vi "FileLoad.vi"(7 "측정거리":dbl, 8 "노이즈 수량":u16=280, 9 "거리 해상도":sgl, 10 "스톡스 데이터 경로 문자열":string, 11 "안티스톡스 데이터 경로 문자열":string) -> (0 "스톡스 인덱스":i32, 1 "안티스톡스 인덱스":i32, 2 "스톡스 배열":dbl[](array[numeric]) caption="스톡스 데이터 배열", 3 "안티스톡스 배열":dbl[](array[numeric]) caption="안티스톡스 데이터 배열", 4 "거리축 배열":dbl[](array[numeric]), 5 "데이터 총량":u32, 6 "대기중":bool)   [LabVIEW 2020]
uses:
  <vilib>/Utility/error.llb/DialogType.ctl
panel:
  out "안티스톡스 OffSet":bool
  out "스톡스 OffSet":bool
  out "안티스톡스 OffSet 평균":dbl
  out "스톡스 OffSet 평균":dbl
  out "OffSet 평균":bool
  out "안티스톡스 읽기 완료":bool caption="읽기완료"
  out "안티스톡스 데이터 경로":path
  out "스톡스 읽기 완료":bool caption="읽기완료"
  out "스톡스 데이터 경로":path
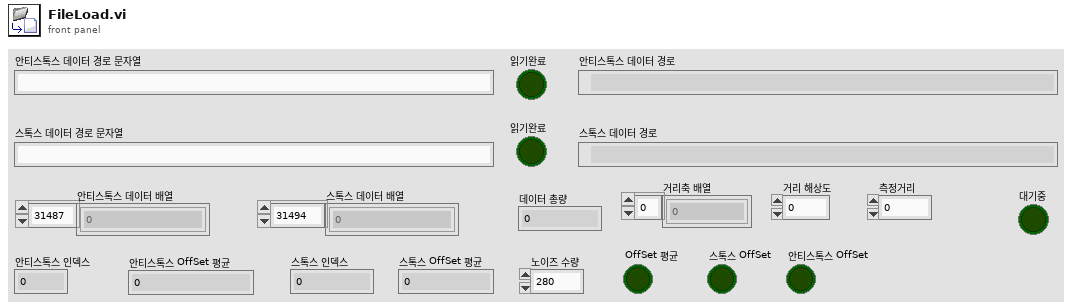
[diagram p1: front panel]
types:
  T1 = typedef "DialogType.ctl" = u16
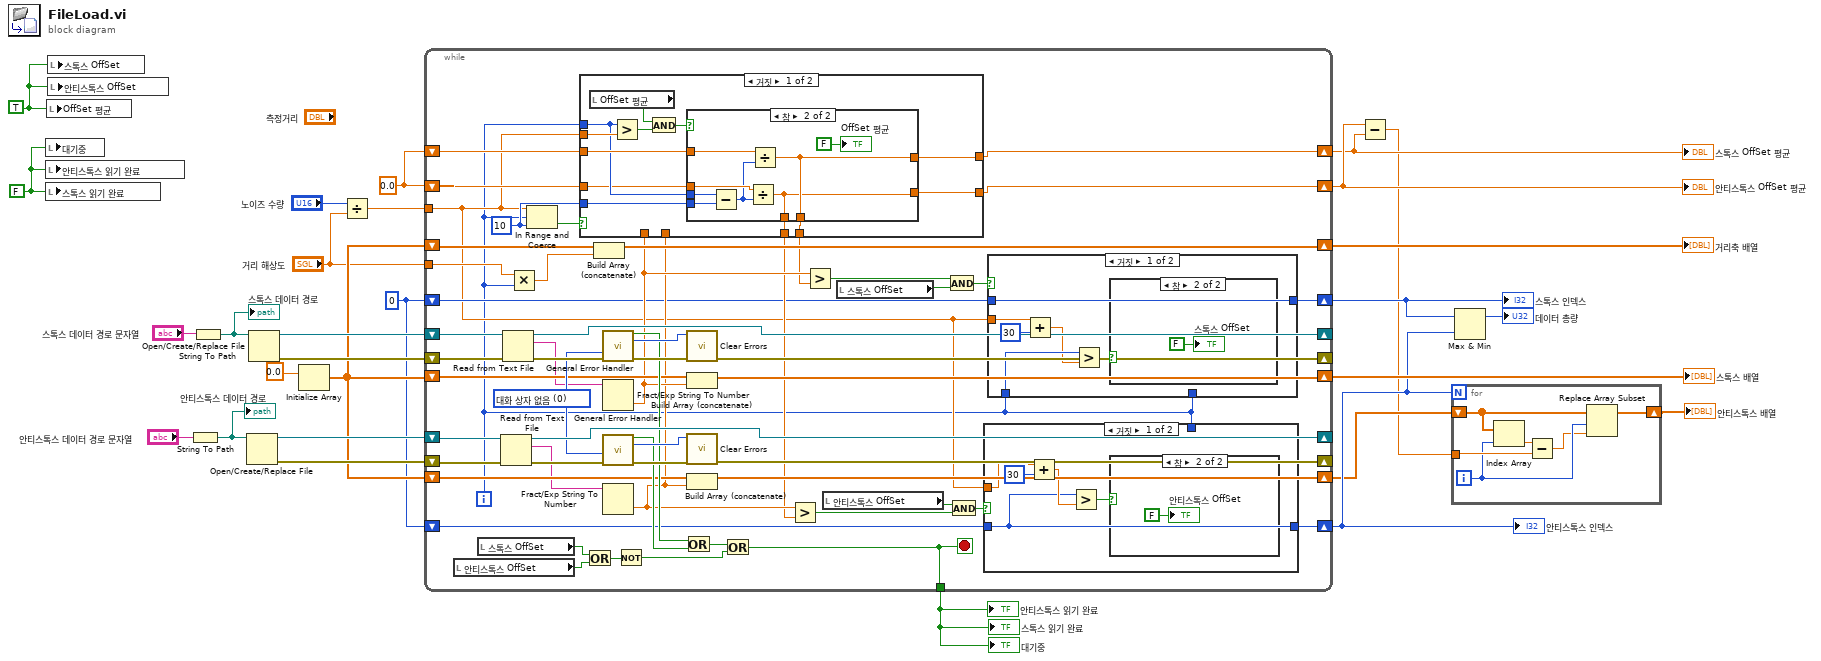
[diagram p0: block diagram]
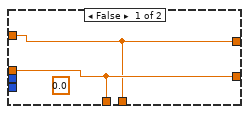
[diagram p6: hidden frame]
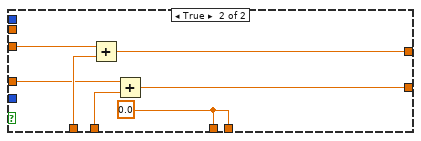
[diagram p7: hidden frame]
diagram:
  w13 = 0
  w12 = TRUE
  w14 = 0.0
  w15 = FALSE
  n1 = local write "대기중"(w15) -> ()
  n2 = local write "안티스톡스 읽기 완료"(w15) -> ()
  n3 = local write "스톡스 읽기 완료"(w15) -> ()
  n4 = local write "OffSet 평균"(w12) -> ()
  n5 = local write "스톡스 OffSet"(w12) -> ()
  n6 = local write "안티스톡스 OffSet"(w12) -> ()
  n7 = String To Path(string="안티스톡스 데이터 경로 문자열") -> (path=w23:path)
  "안티스톡스 데이터 경로" <- w23
  n8 = String To Path(string="스톡스 데이터 경로 문자열") -> (path=w24:path)
  "스톡스 데이터 경로" <- w24
  n9 = Open/Create/Replace File(file path (use dialog)=w23) -> (refnum out=w26:refnum<file>, error out=w25:errorcluster)  [unwired: 5 in, 1 out]
  n10 = Open/Create/Replace File(file path (use dialog)=w24) -> (refnum out=w28:refnum<file>, error out=w27:errorcluster)  [unwired: 5 in, 1 out]
  n11 = Initialize Array(0.0) -> (w17:dbl[])  [unwired: 1 in]
  n12 = Divide(x="노이즈 수량", y="거리 해상도") -> (x/y=w1:sgl)
  n13 = while {
    shift-right: [w78] -> _
    shift-left: w28 -> [w83]
    shift-right: [w79] -> _
    shift-left: w27 -> [w82]
    shift-right: [w70] -> _
    shift-left: w26 -> [w75]
    shift-right: [w71] -> _
    shift-left: w25 -> [w74]
    tunnel: [w30] -> w20
    shift-right: [w63] -> w18
    shift-left: w17 -> [w66]
    shift-right: [w64] -> w6
    shift-left: w17 -> [w65]
    tunnel: "거리 해상도" -> [w60]
    shift-right: [w58] -> w16
    shift-left: w17 -> [w59]
    tunnel: w1 -> [w37]
    shift-right: [w51] -> w9
    shift-left: w14 -> [w53]
    shift-right: [w54] -> w8
    shift-left: w14 -> [w56]
    shift-right: [w47] -> w11
    shift-left: w13 -> [w46]
    shift-right: [w44] -> w7
    shift-left: w13 -> [w45]
    i -> [w36]
    stop <- w30 stop-if-true
    w50 = 10 ("하위 리미트")
    w69 = T1 0 items=["대화 상자 없음", "확인 메시지", "메시지 지속 또는 정지", "확인 메시지 + 경고", "지속/정지 + 경고"] ("type of dialog (OK msg:1)")
    n14 = local read "안티스톡스 OffSet"() -> (w34:bool)
    n15 = local read "스톡스 OffSet"() -> (w35:bool)
    n16 = Read from Text File(file (use dialog)=w75, error in=w74) -> (refnum out=w70:refnum<file>, text=w61:string, error out=w73:errorcluster)  [unwired: 2 in, 1 out]
    n17 = Read from Text File(file (use dialog)=w83, error in=w82) -> (refnum out=w78:refnum<file>, text=w62:string, error out=w80:errorcluster)  [unwired: 2 in, 1 out]
    n18 = Multiply(x=w60, y=w36) -> (x*y=w29:sgl)
    n19 = In Range and Coerce(upper limit=w37, x=w36, lower limit=w50) -> (In Range?=w57:bool)  [unwired: 1 out]
    n20 = Or(x=w35, y=w34) -> (x .or. y?=w33:bool)
    n21 = Build Array (concatenate)(w59, w29) -> (w58:dbl[])
    n22 = call <vilib>:"General Error Handler.vi"("type of dialog (OK msg:1)"=w69, "error in (no error)"=w80) -> ("error?"=w68:bool, "code out"=w81:i32, "error out"=w77:errorcluster)  [unwired: 9 in, 2 out]
    n23 = Fract/Exp String To Number(string=w62) -> (number=w55:dbl)  [unwired: 3 in, 1 out]
    n24 = call <vilib>:"General Error Handler.vi"("type of dialog (OK msg:1)"=w69, "error in (no error)"=w73) -> ("error?"=w67:bool, "code out"=w76:i32, "error out"=w72:errorcluster)  [unwired: 9 in, 2 out]
    n25 = Fract/Exp String To Number(string=w61) -> (number=w52:dbl)  [unwired: 3 in, 1 out]
    n26 = case shown="거짓" w57 {
      tunnel: w56 -> [w109 w127]
      tunnel: w55 -> [_ w126]
      tunnel: [w103 w125] -> w54
      tunnel: w53 -> [w105 w124]
      tunnel: w52 -> [_ w123]
      tunnel: [w102 w122] -> w51
      tunnel: w36 -> [w108 _]
      tunnel: w37 -> [w110 _]
      tunnel: w50 -> [w107 _]
      tunnel: [w106 w121] -> w49
      tunnel: [w104 w121] -> w48
      frame False {
        n27 = local read "OffSet 평균"() -> (w99:bool)
        n28 = Greater?(x=w108, y=w110) -> (0:w100:bool)
        n29 = And(x=w99, y=w100) -> (x .and. y?=w101:bool)
        n30 = case shown="참" w101 {
          tunnel: w109 -> [w111 w120]
          tunnel: [w111 w114] -> w103
          tunnel: w108 -> [_ w119]
          tunnel: w107 -> [_ w118]
          tunnel: [w111 w114] -> w106
          tunnel: w105 -> [w112 w117]
          tunnel: [w112 w113] -> w104
          tunnel: [w112 w113] -> w102
          frame False {
            (unwired) 0.0
          }
          frame True {
            n31 = Subtract(x=w119, y=w118) -> (x-y=w116:i32)
            n32 = Divide(x=w117, y=w116) -> (x/y=w113:dbl)
            n33 = Divide(x=w120, y=w116) -> (x/y=w114:dbl)
            "OffSet 평균" <- FALSE
          }
        }
      }
      frame True {
        w121 = 0.0
        n34 = Add(x=w127, y=w126) -> (x+y=w125:dbl)
        n35 = Add(x=w124, y=w123) -> (x+y=w122:dbl)
      }
    }
    n36 = Not(x=w33) -> (.not. x?=w31:bool)
    n37 = Or(x=w68, y=w67) -> (x .or. y?=w32:bool)
    n38 = call <vilib>:"Clear Errors.vi"("error in (no error)"=w77, "specific error code to clear (0: all)"=w81) -> ("error out"=w79:errorcluster)  [unwired: 4 in, 1 out]
    n39 = Build Array (concatenate)(w66, w55) -> (w63:dbl[])
    n40 = call <vilib>:"Clear Errors.vi"("error in (no error)"=w72, "specific error code to clear (0: all)"=w76) -> ("error out"=w71:errorcluster)  [unwired: 4 in, 1 out]
    n41 = Build Array (concatenate)(w65, w52) -> (w64:dbl[])
    n42 = Or(x=w32, y=w31) -> (x .or. y?=w30:bool)
    n43 = Greater?(x=w52, y=w48) -> (0:w39:bool)
    n44 = Greater?(x=w55, y=w49) -> (0:w43:bool)
    n45 = local read "안티스톡스 OffSet"() -> (w38:bool)
    n46 = local read "스톡스 OffSet"() -> (w41:bool)
    n47 = And(x=w43, y=w41) -> (x .and. y?=w42:bool)
    n48 = And(x=w38, y=w39) -> (x .and. y?=w40:bool)
    n49 = case shown="거짓" w40 {
      tunnel: [w86 w90] -> w44
      tunnel: w45 -> [w86 _]
      tunnel: w36 -> [_ w90]
      tunnel: w37 -> [w85 _]
      frame False {
        n50 = Add(x=w85, y=u16 30) -> (x+y=w87:sgl)
        n51 = Greater?(x=w86, y=w87) -> (0:w84:bool)
        n52 = case shown="참" w84 {
          frame False {
          }
          frame True {
            "안티스톡스 OffSet" <- FALSE ("안티스톡스 노이즈")
          }
        }
      }
      frame True {
      }
    }
    n53 = case shown="거짓" w42 {
      tunnel: [w96 w98] -> w47
      tunnel: w46 -> [w96 _]
      tunnel: w36 -> [_ w98]
      tunnel: w37 -> [w93 _]
      tunnel: w36 -> [w94 _]
      frame False {
        n54 = Add(x=w93, y=u16 30) -> (x+y=w91:sgl)
        n55 = Greater?(x=w94, y=w91) -> (0:w95:bool)
        n56 = case shown="참" w95 {
          frame False {
          }
          frame True {
            "스톡스 OffSet" <- FALSE ("스톡스 노이즈")
          }
        }
      }
      frame True {
      }
    }
  }
  "대기중" <- w20
  "스톡스 읽기 완료" <- w20
  "안티스톡스 읽기 완료" <- w20
  "스톡스 배열" <- w18
  "스톡스 인덱스" <- w11
  "거리축 배열" <- w16
  "안티스톡스 인덱스" <- w7
  "스톡스 OffSet 평균" <- w8
  "안티스톡스 OffSet 평균" <- w9
  n57 = Subtract(x=w9, y=w8) -> (x-y=w5:dbl)
  n58 = for {
    N: w7 -> [_]
    shift-right: [w130] -> w4
    shift-left: w6 -> [w131]
    tunnel: w5 -> [w132]
    i -> [w129]
    n59 = Index Array(array=w131, index=w129) -> (element=w133:dbl)
    n60 = Subtract(x=w133, y=w132) -> (x-y=w128:dbl)
    n61 = Replace Array Subset(array=w131, new element=w128, index=w129) -> (w130:dbl[])
  }
  "안티스톡스 배열" <- w4
  n62 = Max & Min(x=w11, y=w7) -> (max(x,y)=→"데이터 총량":i32)  [unwired: 1 out]
